vi "UsrProfiles-Load user profile-All values.vi"(8 "error in":errorcluster) -> (0 "error out":errorcluster)   [LabVIEW 2013]
uses:
  Typedefs/Save-Load enum.ctl
  Typedefs/Which path.ctl
  Typedefs/HW config states enum.ctl
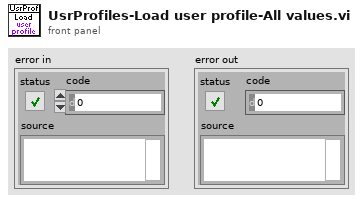
[diagram p1: front panel]
types:
  T1 = typedef "HW config states enum.ctl" = enum16{"Load from file", "Save to file", "Write all", "Read all", "Write XY stage settings", "Write DAQ FPGA settings", "Write Control FPGA settings", "Write Phys Channels", "Clear", "Compare from file"}
  T2 = typedef "Which path.ctl" = enum16{"Configuration Files", "Calibration Files", "Images", "Setup.ini", "Loaded User profile.ini", "User's-Previous session.ini", "New user profile.ini", "Selected User profile.ini", "User profiles folder", "Power meter scaling.txt", "FOV Cal.ini"}
  T3 = typedef "Save-Load enum.ctl" = enum16{"Save to file", "Load from file", "Compare from file"}
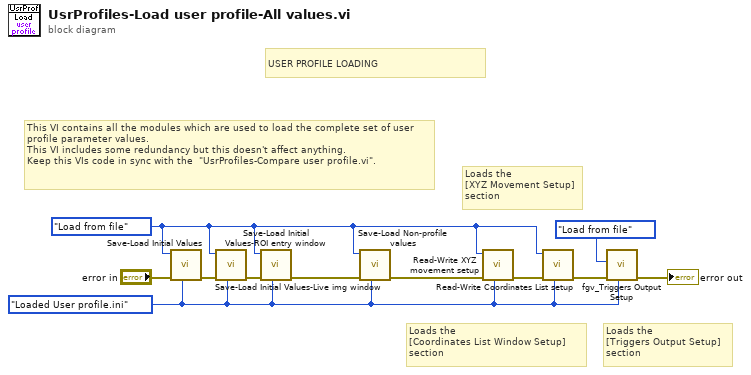
[diagram p0: block diagram]
diagram:
  w2 = Which_path."Loaded User profile.ini" ("Which file?")
  w6 = Save-Load_enum."Load from file" ("Function")
  # "USER PROFILE LOADING"
  # "Loads the\n[Triggers Output Setup]\nsection"
  # "Loads the\n[Coordinates List Window Setup]\nsection"
  # "Loads the\n[XYZ Movement Setup]\nsection"
  # "This VI contains all the modules which are used to load the complete set of user profile parameter values.\nThis VI includes some redundancy but this doesn't affect anything.\nKeep this VIs code in sync with the  \"UsrProfiles-Compare user profile.vi\"."
  n1 = call "Save-Load Initial Values.vi"("Which file? (User profile.ini)"=w2, "error in"="error in", "Function"=w6) -> ("error out"=w10:errorcluster)  [unwired: 8 in]
  n2 = call "Save-Load Initial Values-Live img window.vi"("Which file? (User profile.ini)"=w2, "error in"=w10, "Function"=w6) -> ("error out"=w11:errorcluster)  [unwired: 8 in]
  n3 = call "Save-Load Initial Values-ROI entry window.vi"("Which file? (User profile.ini)"=w2, "error in"=w11, "Function"=w6) -> ("error out"=w1:errorcluster)  [unwired: 8 in]
  n4 = call "Save-Load Non-profile values.vi"("Which file? (User profile.ini)"=w2, "error in"=w1, "Function"=w6) -> ("error out"=w7:errorcluster)  [unwired: 8 in]
  n5 = call "Read-Write XYZ movement setup.vi"("Which file? (User profile.ini)"=w2, "error in"=w7, "Function"=w6) -> ("error out"=w8:errorcluster)  [unwired: 8 in]
  n6 = call "Read-Write Coordinates List setup.vi"("Which file?"=w2, "error in"=w8, "Function"=w6) -> ("error out"=w5:errorcluster)  [unwired: 8 in]
  n7 = call "fgv_Triggers Output Setup.vi"("Which file? (User profile.ini)"=w2, "error in (no error)"=w5, "Function"=HW_config_states_enum."Load from file") -> ("error out"=→"error out":errorcluster)  [unwired: 7 in, 1 out]
